vi "Get Tests Events by Test ID.vi"(8 "error in (no error)":errorcluster, 10 "Test ID":string, 11 "Test Event Storage in":refnum<class "Test Event Storage.lvclass">) -> (0 "error out":errorcluster, 2 "Test Events":T1[](array[typedef]), 3 "Test Event Storage out":refnum<class "Test Event Storage.lvclass">)   [LabVIEW 2013, in "Caraya.lvlib" / "Test Event Storage.lvclass"]
uses:
  Test Event Storage.lvclass
  Test Result/Assert Event Data.ctl
  Test Event Storage.lvclass/Test Event Storage.ctl
  Test Result/Test Result.lvclass
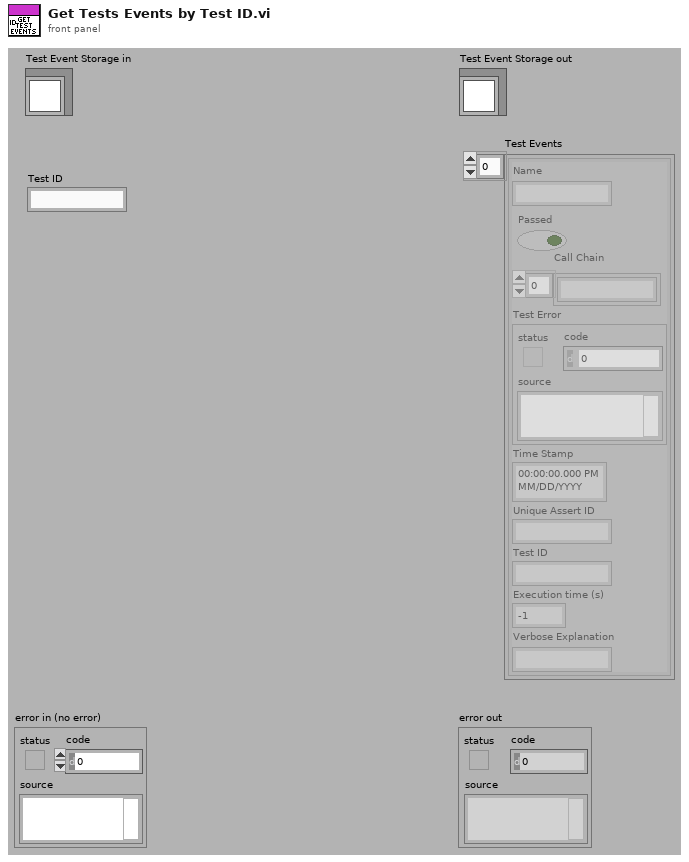
[diagram p1: front panel]
types:
  T1 = typedef "Caraya.lvlib/Test Result.lvclass/Assert Event Data.ctl" = cluster{"Name":string, "Passed":bool, "Call Chain":string[], "Test Error":errorcluster, "Time Stamp":timestamp, "Unique Assert ID":string, "Test ID":string, "Execution time (s)":dbl, "Verbose Explanation":string}
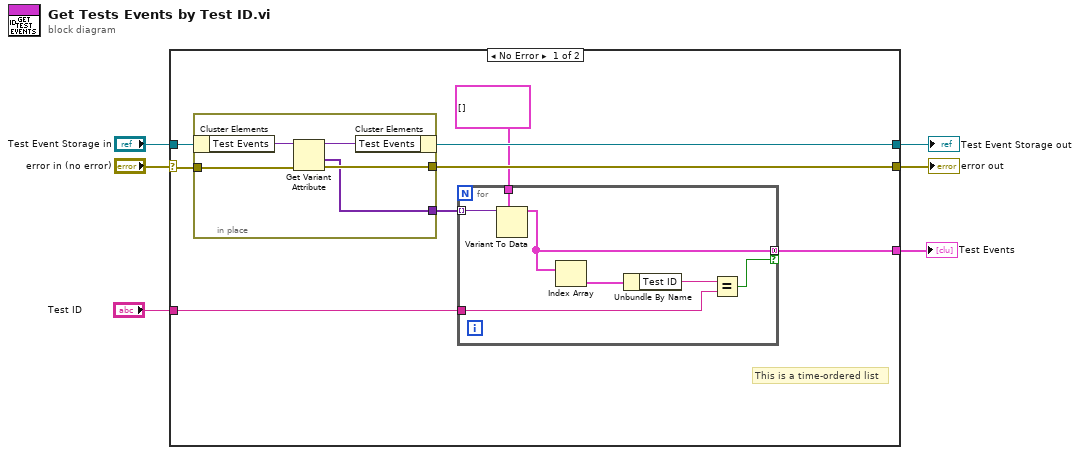
[diagram p0: block diagram]
diagram:
  n1 = case shown="No Error" "error in (no error)" {
    selector: "error in (no error)" -> [w11 w28]
    tunnel: [w14 w28] -> w5
    tunnel: [w13 w27] -> w3
    tunnel: "Test Event Storage in" -> [w12 w27]
    tunnel: [w9 _] -> w2
    tunnel: "Test ID" -> [w10 _]
    frame No Error {
      # "This is a time-ordered list"
      n2 = in-place {
        in-place-border: w11 -> [w25]
        in-place-border: [w23] -> w14
        in-place-border: [w22] -> w7
        n3 = in-place-cluster #1(w12) -> ("Test Events"=w26:variant)
        n4 = Get Variant Attribute(Variant=w26, error in=w25) -> (duplicate Variant=w24:variant, values=w22:variant[], error out=w23:errorcluster)  [unwired: 2 in, 1 out]
        n5 = in-place-cluster #1("Test Events"=w24) -> (w13:refnum<class "Test Event Storage.lvclass">)
      }
      n6 = for {
        tunnel: w10 -> [w20]
        tunnel: [w16] -> w9 mode=concatenating if=w19
        tunnel: T1[] [] -> [w18]
        tunnel: w7 -> [w17] mode=indexing
        n7 = Variant To Data(type=w18, Variant=w17) -> (data=w16:T1[])  [unwired: 1 in, 1 out]
        n8 = Index Array(array=w16) -> (element=w15:T1)  [unwired: 1 in]
        n9 = Unbundle By Name(w15) -> ("Test ID"=w21:string)
        n10 = Equal?(x=w21, y=w20) -> (x = y?=w19:bool)
      }
    }
    frame Error {
    }
  }
  "error out" <- w5
  "Test Event Storage out" <- w3
  "Test Events" <- w2
